vi "Extract8BitImage.vi"(2 "Flip?":bool, 3 "Image in":T1 {"Dialogs" format="%.0b"}) -> (0 "Intensity Graph":u8[][](graph), 1 "Image out":T1 {"Dialogs" format="%.0b"})   [LabVIEW 2014]
uses:
  QT_Image.ctl
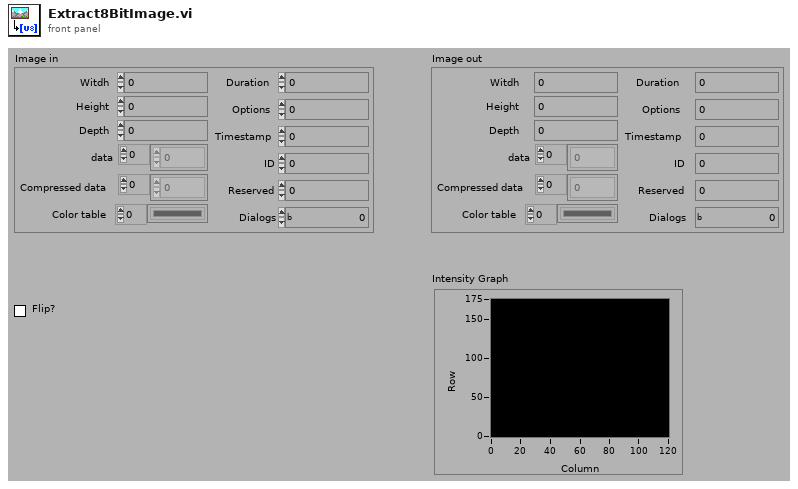
[diagram p1: front panel]
types:
  T1 = typedef "QT_Image.ctl" = cluster{"Witdh":i32, "Height":i32, "Depth":i32, "data":u8[], "Compressed data":u8[], "Color table":u32[], "Duration":i32, "Options":i32, "Timestamp":i32, "ID":i32, "Reserved":i32, "Dialogs":u32}
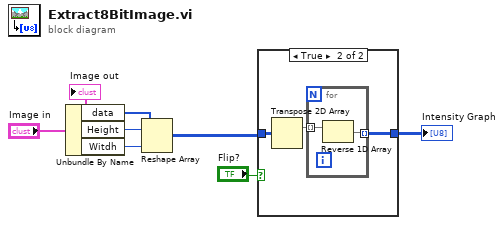
[diagram p0: block diagram]
diagram:
  n1 = Unbundle By Name("Image in") -> ("data"=w5:u8[], "Height"=w7:i32, "Witdh"=w6:i32)
  n2 = Reshape Array(w5, w7, w6) -> (w3:u8[][])
  n3 = case shown="True" "Flip?" {
    tunnel: w3 -> [w8 w11]
    tunnel: [w8 w9] -> w2
    frame False {
    }
    frame True {
      n4 = Transpose 2D Array(2D array=w11) -> (transposed array=w10:u8[][])
      n5 = for {
        tunnel: w10 -> [w13] mode=indexing
        tunnel: [w12] -> w9 mode=indexing
        n6 = Reverse 1D Array(array=w13) -> (reversed array=w12:u8[])
      }
    }
  }
  "Intensity Graph" <- w2
  "Image out" <- "Image in"
